vi "Read UDP.vi"(8 "error in (no error)":errorcluster, 9 "Timeout (ms)":i32=100, 10 "Max Size":i32=2048, 11 "UDP in":refnum<class "UDP.lvclass">) -> (0 "error out":errorcluster, 2 "String":string, 3 "UDP out":refnum<class "UDP.lvclass">)   [LabVIEW 2018, in "UDP.lvlib" / "UDP.lvclass"]
uses:
  UDP.lvclass
  UDP.lvclass/UDP.ctl
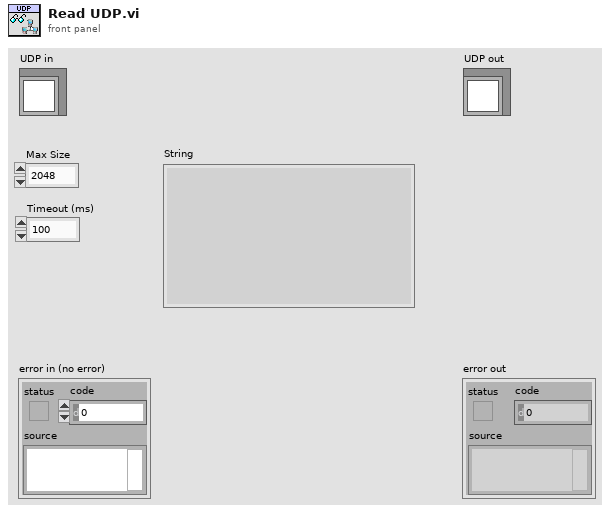
[diagram p1: front panel]
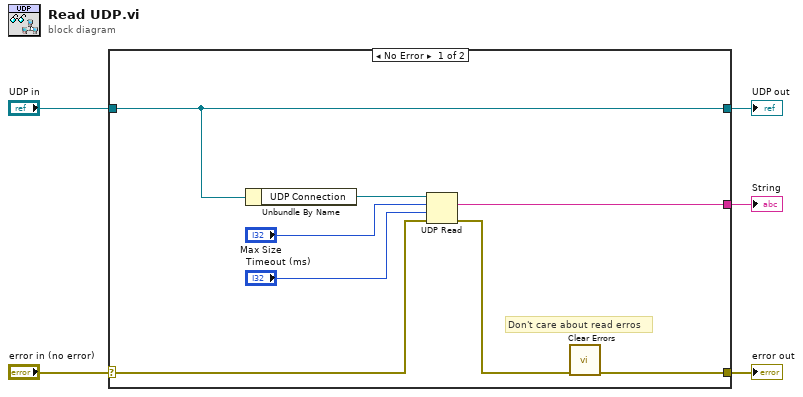
[diagram p0: block diagram]
diagram:
  n1 = case shown="No Error" "error in (no error)" {
    selector: "error in (no error)" -> [w8 w15]
    tunnel: [w6 w15] -> w4
    tunnel: [w13 w14] -> w2
    tunnel: "UDP in" -> [w13 w14]
    tunnel: [w9 _] -> w1
    frame No Error {
      # "Don't care about read erros"
      n2 = Unbundle By Name(w13) -> ("UDP Connection"=w12:refnum<k16>)
      n3 = UDP Read(connection ID=w12, max size (548)="Max Size", timeout ms (25000)="Timeout (ms)", 8:w8) -> (data out=w9:string, error out=w7:errorcluster)  [unwired: 3 out]
      n4 = call <vilib>:"Clear Errors.vi"("error in (no error)"=w7) -> ("error out"=w6:errorcluster)  [unwired: 5 in, 1 out]
    }
    frame Error {
    }
  }
  "error out" <- w4
  "UDP out" <- w2
  "String" <- w1
